vi "Unsubscribe (Async).vi"(9 "Topic":string, 10 "error in (no error)":errorcluster, 11 "WAMP Client in":refnum<class "WAMP Client.lvclass">) -> (1 "Result Event":refnum<user-event>, 2 "error out":errorcluster, 3 "WAMP Client out":refnum<class "WAMP Client.lvclass">)   [LabVIEW 2020, in "WAMP Client.lvclass"]
uses:
  <userlib>/wamplv/WAMP Client/WAMP Client.lvclass
  <userlib>/wamplv/WAMP Client/TypeDef/UNSUBSCRIBE Result.ctl
  <userlib>/wamplv/WAMP Client/TypeDef/UNSUBSCRIBE Request Data.ctl
  <userlib>/wamplv/WAMP Client/TypeDef/Internal Message Type.ctl
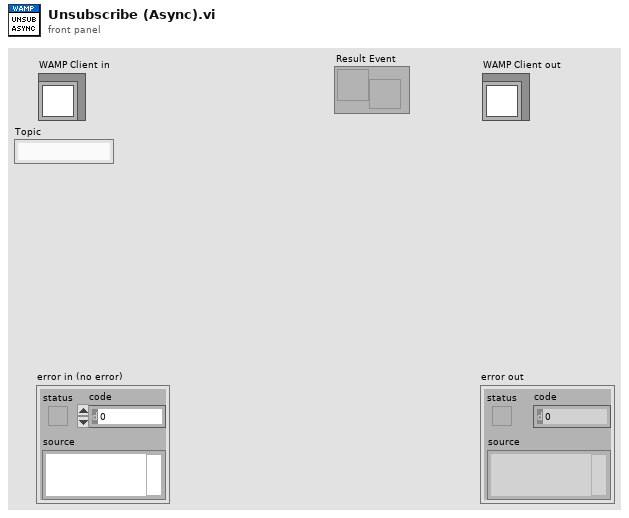
[diagram p1: front panel]
types:
  T1 = typedef "WAMP Client.lvclass/Internal Message Type.ctl" = enum16{"Subscribe", "Handle Subscribed", "Handle Event", "Unsubscribe", "Handle Unsubscribed", "Publish", "Handled Published", "Goodbye", "Handle Goodbye", "Call", "Handle Result", "Register", "Handle Registered", "Unregister", "Handle Unregistered", "Handle Invocation", "Yield"}
  T2 = typedef "WAMP Client.lvclass/UNSUBSCRIBE Request Data.ctl" = cluster{"Topic":string, "Unsubscribe Result Received Event":refnum<user-event>}
  T3 = typedef "WAMP Client.lvclass/UNSUBSCRIBE Result.ctl" = cluster{"Success?":bool, "Error":errorcluster}
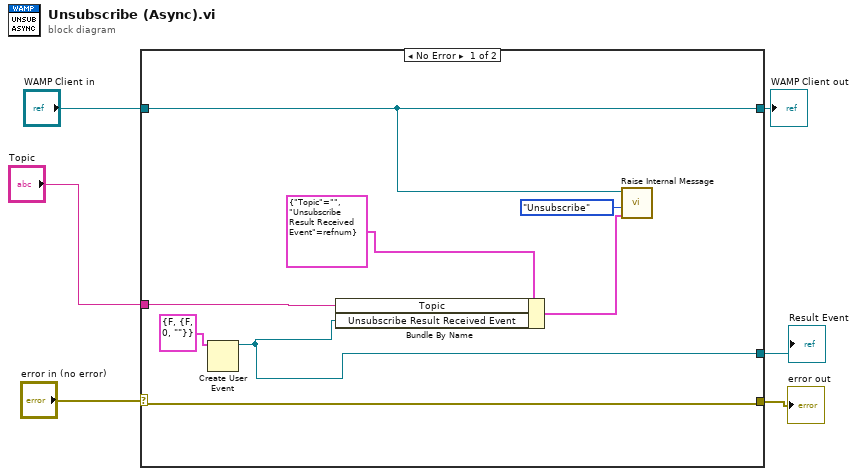
[diagram p0: block diagram]
diagram:
  n1 = case shown="No Error" "error in (no error)" {
    selector: "error in (no error)" -> [w14 w16]
    tunnel: [w14 w16] -> w5
    tunnel: [w13 w15] -> w3
    tunnel: "WAMP Client in" -> [w13 w15]
    tunnel: [w8 _] -> w1
    tunnel: "Topic" -> [w11 _]
    frame No Error {
      n2 = Create User Event(user event datatype=T3 {"Success?"=FALSE, "Error"={"status"=FALSE, "code"=0, "source"=""}} ("Subcsribe Result")) -> (user event=w8:refnum<user-event>)  [unwired: 1 in, 1 out]
      n3 = Bundle By Name(cluster=T2 {"Topic"="", "Unsubscribe Result Received Event"=refnum} ("Cluster"), "Topic"=w11, "Unsubscribe Result Received Event"=w8) -> (w12:T2)
      n4 = call-dynamic "Raise Internal Message.vi"("Variant"=w12, "Internal Message Type"=Internal_Message_Type."Unsubscribe", "WAMP Client in"=w13) -> ()  [unwired: 7 in, 2 out]
    }
    frame Error {
    }
  }
  "error out" <- w5
  "WAMP Client out" <- w3
  "Result Event" <- w1
